vi "HWIO config.vi"(8 "error in":errorcluster) -> (0 "error out":errorcluster)   [LabVIEW 2015]
uses:
  Control Button/Save.ctl
panel:
  in  "Save":T1
  in  "Exit":bool
  in  "HWIO Configuration List":string[][](table)
  # "Hardware input & Output"
  # "Control Button"
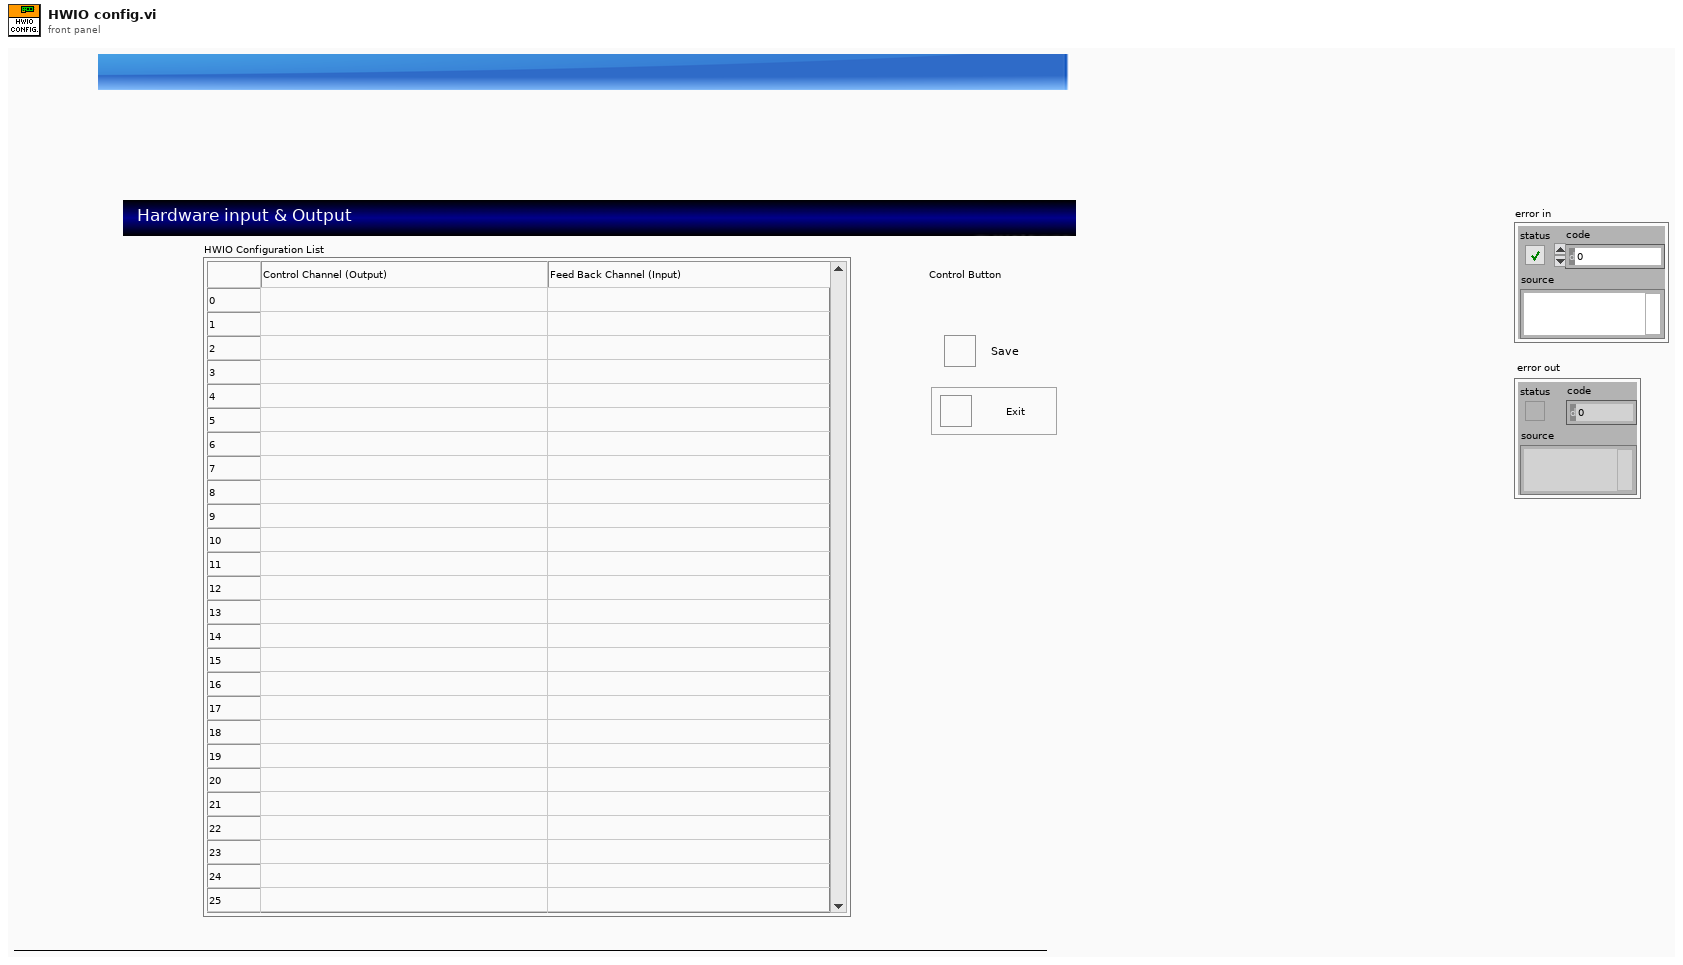
[diagram p1: front panel]
types:
  T1 = typedef "Save.ctl" = bool
  T2 = enum16{"Selection", "Insert Data", "Edit", "Read"}
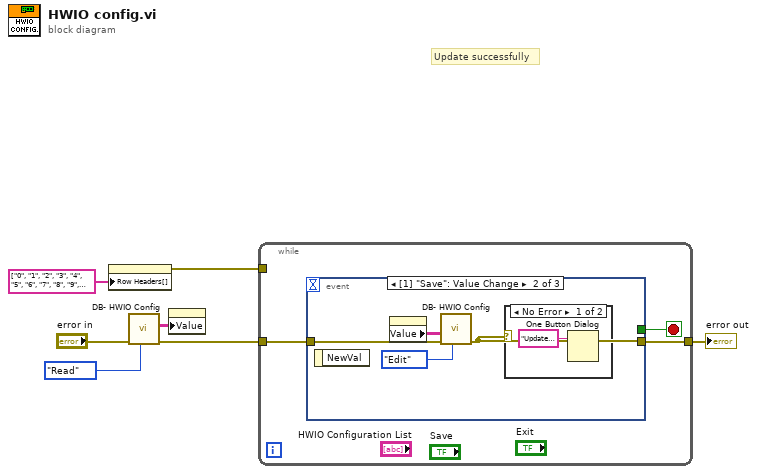
[diagram p0: block diagram]
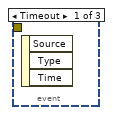
[diagram p2: hidden frame]
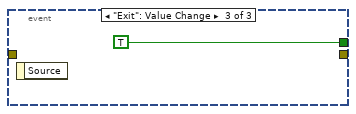
[diagram p4: hidden frame]
diagram:
  # "Update successfully"
  n1 = property on="HWIO Configuration List" class="Tbl (strict)"("Row Headers[]"=string[] ["0", "1", "2", "3", "4", "5", "6", "7", "8", "9", "10", "11", "12", "13", "14", "15", "16", "17", "18", "19", "20", "21", "22", "23", "24", "25", "26", "27", "28", "29", "30", "31"] ("Row Header Strings[]")) -> (error out=w5:errorcluster)  [unwired: 2 in, 1 out]
  n2 = call "DB- HWIO Config.vi"("Enum"=T2."Read", "error in (no error)"="error in") -> ("error out"=w3:errorcluster, "Read Databaase"=w2:string[][])  [unwired: 7 in, 1 out]
  n3 = property on="HWIO Configuration List" class="Tbl (strict)"("Value"=w2) -> ()  [unwired: 2 in, 2 out]
  n4 = while {
    tunnel: w3 -> [w8]
    tunnel: [w9] -> w6
    tunnel: w5 -> [_]
    stop <- w10 stop-if-true
    n5 = event shown="[1] \"Save\": Value Change" {
      selector: _ -> [_ _ _]
      dyn-events: _ -> [_ _ _]
      timeout: _ -> [_ _ _]
      tunnel: [_ _ TRUE] -> w10
      tunnel: [_ w11 _] -> w9
      tunnel: w8 -> [_ w12 _]
      event Timeout {
        n6 = event-data() -> ()  [unwired: 1 in, 3 out]
      }
      event Value Change {
        n7 = event-data() -> ()  [unwired: 1 in, 1 out]
        n8 = property on="HWIO Configuration List" class="Tbl (strict)"() -> ("Value"=w13:string[][])  [unwired: 2 in, 2 out]
        n9 = call "DB- HWIO Config.vi"("Enum"=T2."Edit", "error in (no error)"=w12, "Database table"=w13) -> ("error out"=w11:errorcluster)  [unwired: 6 in, 2 out]
        n10 = case shown="No Error" w11 {
          frame No Error {
            n11 = One Button Dialog(message="Update successfully") -> ()  [unwired: 1 in, 1 out]
          }
          frame Error {
          }
        }
      }
      event "Exit": Value Change {
        n12 = event-data() -> ()  [unwired: 1 in, 1 out]
      }
    }
  }
  "error out" <- w6
